vi "save_s2p_file.vi"(8 "button_save_s2p":bool, 10 "data_array_in":dbl[][](array[numeric]), 11 "freq_array_in":dbl[](array[numeric])) -> ()   [LabVIEW 2025]
panel:
  out "Save Buffer":string
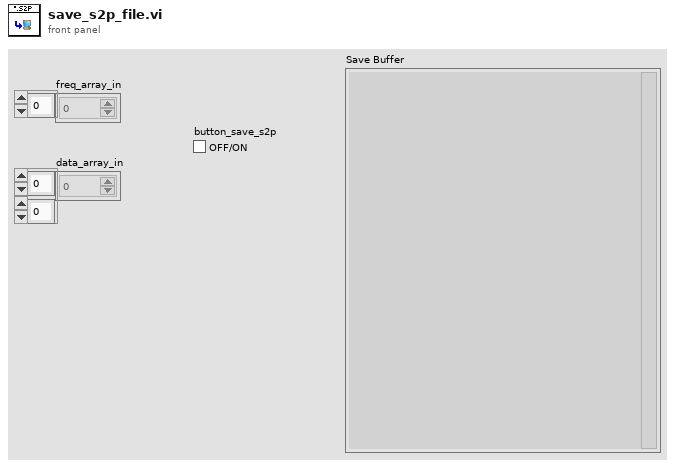
[diagram p1: front panel]
types:
  T1 = enum16{"open", "replace", "create", "open or create", "replace or create", "replace or create with confirmation"}
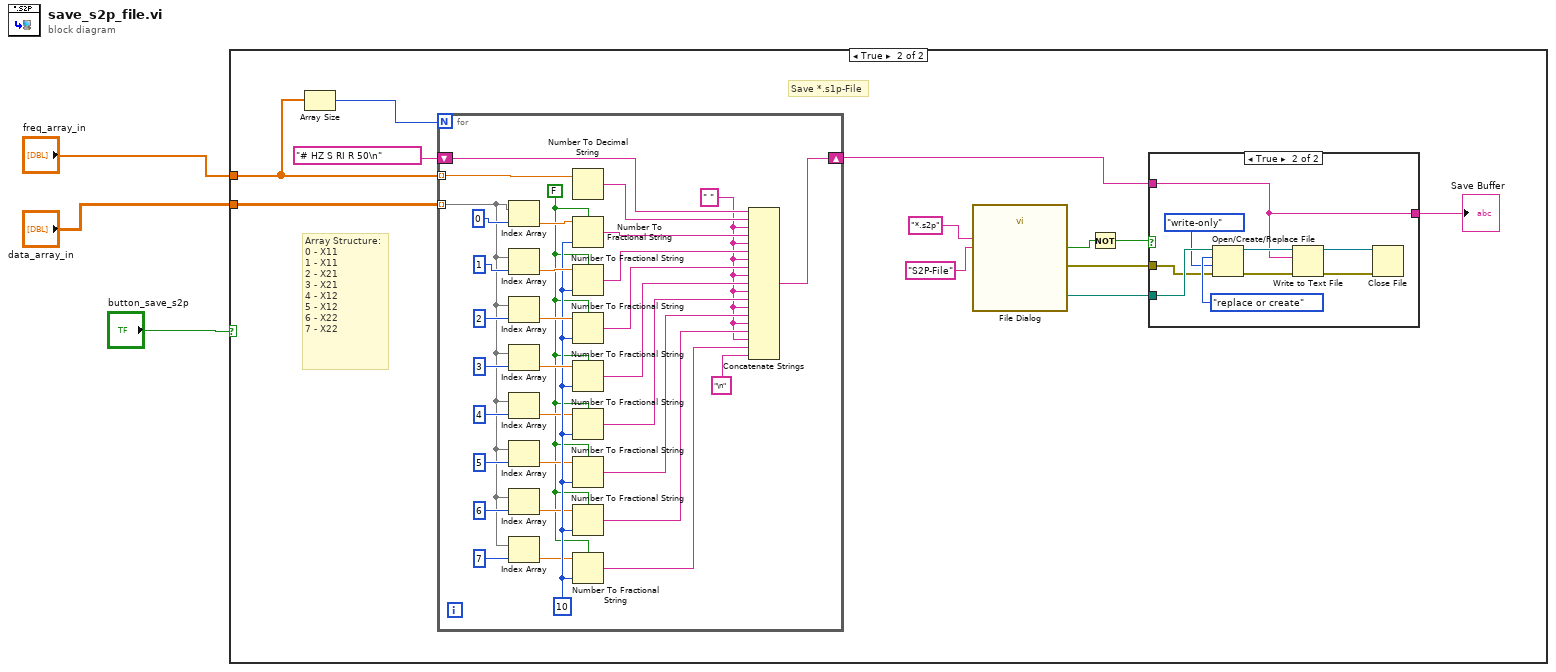
[diagram p0: block diagram]
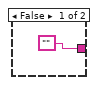
[diagram p3: hidden frame]
diagram:
  n1 = case shown="True" "button_save_s2p" {
    tunnel: "freq_array_in" -> [_ w5]
    tunnel: "data_array_in" -> [_ w14]
    frame False {
    }
    frame True {
      # "Array Structure:\n0 - X11\n1 - X11\n2 - X21\n3 - X21\n4 - X12\n5 - X12\n6 - X22\n7 - X22"
      # "Save *.s1p-File"
      n2 = Array Size(array=w5) -> (size(s)=w4:i32)
      n3 = for {
        N: w4 -> [_]
        shift-right: [w51] -> w9
        shift-left: "# HZ S RI R 50\n" -> [w50]
        tunnel: w5 -> [w49] mode=indexing
        tunnel: w14 -> [w38] mode=indexing
        w37 = i16 10 ("precision (6)")
        w26 = FALSE ("use system decimal point (T)")
        w29 = " " ("string")
        n4 = Index Array(array=w38, index=0 ("index (col)")) -> (element=w55:dbl)
        n5 = Index Array(array=w38, index=1 ("index (col)")) -> (element=w53:dbl)
        n6 = Index Array(array=w38, index=2 ("index (col)")) -> (element=w46:dbl)
        n7 = Index Array(array=w38, index=3 ("index (col)")) -> (element=w45:dbl)
        n8 = Index Array(array=w38, index=4 ("index (col)")) -> (element=w36:dbl)
        n9 = Index Array(array=w38, index=5 ("index (col)")) -> (element=w35:dbl)
        n10 = Index Array(array=w38, index=6 ("index (col)")) -> (element=w34:dbl)
        n11 = Index Array(array=w38, index=7 ("index (col)")) -> (element=w33:dbl)
        n12 = Number To Decimal String(number=w49) -> (decimal integer string=w56:string)  [unwired: 1 in]
        n13 = Number To Fractional String(use system decimal point (T)=w26, number=w55, precision (6)=w37) -> (F-format string=w54:string)  [unwired: 1 in]
        n14 = Number To Fractional String(use system decimal point (T)=w26, number=w53, precision (6)=w37) -> (F-format string=w52:string)  [unwired: 1 in]
        n15 = Number To Fractional String(use system decimal point (T)=w26, number=w46, precision (6)=w37) -> (F-format string=w44:string)  [unwired: 1 in]
        n16 = Number To Fractional String(use system decimal point (T)=w26, number=w45, precision (6)=w37) -> (F-format string=w43:string)  [unwired: 1 in]
        n17 = Number To Fractional String(use system decimal point (T)=w26, number=w36, precision (6)=w37) -> (F-format string=w32:string)  [unwired: 1 in]
        n18 = Number To Fractional String(use system decimal point (T)=w26, number=w35, precision (6)=w37) -> (F-format string=w31:string)  [unwired: 1 in]
        n19 = Number To Fractional String(use system decimal point (T)=w26, number=w34, precision (6)=w37) -> (F-format string=w30:string)  [unwired: 1 in]
        n20 = Number To Fractional String(use system decimal point (T)=w26, number=w33, precision (6)=w37) -> (F-format string=w28:string)  [unwired: 1 in]
        n21 = Concatenate Strings(w50, w56, w29, w54, w29, w52, w29, w44, w29, w43, w29, w32, w29, w31, w29, w30, w29, w28, "\n" ("string")) -> (w51:string)
      }
      n22 = call "File Dialog"("pattern (all files)"="*.s2p" ("pattern label"), "pattern label"="S2P-File") -> ("selected path"=w11:path, "cancelled"=w7:bool, "error out"=w10:errorcluster)  [unwired: 10 in, 1 out]
      n23 = Not(x=w7) -> (.not. x?=w8:bool)
      n24 = case shown="True" w8 {
        tunnel: w11 -> [_ w24]
        tunnel: w10 -> [_ w23]
        tunnel: w9 -> [_ w17]
        tunnel: ["" w17] -> w6
        frame False {
        }
        frame True {
          n25 = Open/Create/Replace File(file path (use dialog)=w24, error in=w23, operation (0:open)=T1."replace or create", access (0:read/write)=enum16{"read/write", "read-only", "write-only"}."write-only") -> (refnum out=w22:refnum<file>, error out=w21:errorcluster)  [unwired: 2 in, 1 out]
          n26 = Write to Text File(file (use dialog)=w22, text=w17, error in=w21) -> (refnum out=w19:refnum<file>, error out=w20:errorcluster)  [unwired: 1 in, 1 out]
          n27 = Close File(refnum=w19, error in=w20) -> ()  [unwired: 2 out]
        }
      }
      "Save Buffer" <- w6
    }
  }
